vi "BellaBeamLine.vi"() -> ()   [LabVIEW 2020]
uses:
  StagingBeamline/Controls/eventtypdef1.ctl
  Shared/GUI_Template/GUI_master/tcp new data cluster.ctl
  Device Drivers/LEPS Interface/Filter_typdef.ctl
panel:
  in  "filter.var 2::15":T1=enum."OD1" caption="Filter Wheel"
  in  "filter.var 4::15":T1=enum."OD1" caption="Filter Wheel"
  in  "filter.var 5::15":T1=enum."OD1" caption="Filter Wheel"
  in  "filter.var 1::15":T1=enum."OD1" caption="Filter Wheel"
  in  "GUIdevice 15":string="71146 LEPS Interface"
  in  "stepsize::14":dbl=0.001 caption="Step Size" min=0.0 max=1.0 format="%.3f"
  in  "stepsize::12":dbl=0.001 caption="Step Size" min=0.0 max=1.0 format="%.3f"
  in  "stepsize::13":dbl=0.001 caption="Step Size" min=0.0 max=1.0 format="%.3f"
  in  "relativeMove.Axis 1pos::14":bool
  in  "relativeMove.Axis 1neg::14":bool
  in  "relativeMove.Axis 3pos::12":bool
  in  "relativeMove.Axis 3neg::12":bool
  in  "GUIdevice 14":string="BELLA_ESP_2"
  in  "relativeMove.Axis 2neg::14":bool
  in  "relativeMove.Axis 2pos::14":bool
  in  "relativeMove.Axis 3pos::14":bool
  in  "relativeMove.Axis 3neg::14":bool
  in  "GUIdevice 12":string="BellaESP"
  in  "relativeMove.Axis 1neg::12":bool
  in  "relativeMove.Axis 1pos::12":bool
  in  "relativeMove.Axis 2pos::12":bool
  in  "relativeMove.Axis 2neg::12":bool
  in  "GUIdevice 13":string="BELLA_ESP_M1"
  in  "relativeMove.Axis 1neg::13":bool
  in  "relativeMove.Axis 1pos::13":bool
  in  "relativeMove.Axis 2pos::13":bool
  in  "relativeMove.Axis 2neg::13":bool
  out "Boolean":bool
  in  "Dutch>>Magnet":bool caption="Mirror"
  out "GUIdevice 11":string="StagingImageLocation"
  out "GUIdevice 10":string="StagingImageLocation"
  out "GUIdevice 9":string="StagingTRA3"
  in  "GUIdevice 8":string="StagingTelescopePosition"
  in  "M5Cam>>Camera":bool caption="M5Cam"
  in  "M4Cam>>Camera":bool caption="M4Cam"
  in  "M2Cam>>Camera":bool caption="M2Cam"
  out "GUIdevice 7":string="StagingDelayStage"
  in  "DeviceControl":bool=TRUE
  in  "ignore interlock::6":bool=TRUE caption="ignore interlock"
  in  "GUIdevice 6":string="StagingInterlock"
  out "fire interlock::6":bool caption="Interlock"
  in  "GUIdevice 5":string="BellaSRS"
  out "fire::5":string
  in  "fire!!!":bool caption="fire"
  in  "Mode::5":bool
  out "GUIdevice 4":string="StagingImageLocation"
  in  "GUIdevice 3":string="StagingFocusPositionBeam2"
  in  "GUIdevice 2":string="StagingFocusPositionBeam1"
  out "XHairs":refnum<vi>[](array[refnum])
  out "device status::1":string="no scan"
  in  "GUIdevice 1":string="Staging1Wire"
  in  "M1Cam>>Camera":bool caption="M1Cam"
  in  "Bella_LP_Mode>>Camera":bool caption="Bella_LP_Mode"
  in  "stop":bool
  # "M5 X-Axis, LP Mode CAMS"
  # "M5 Y-Axis, M4 CAMS"
  # "M2 CAM"
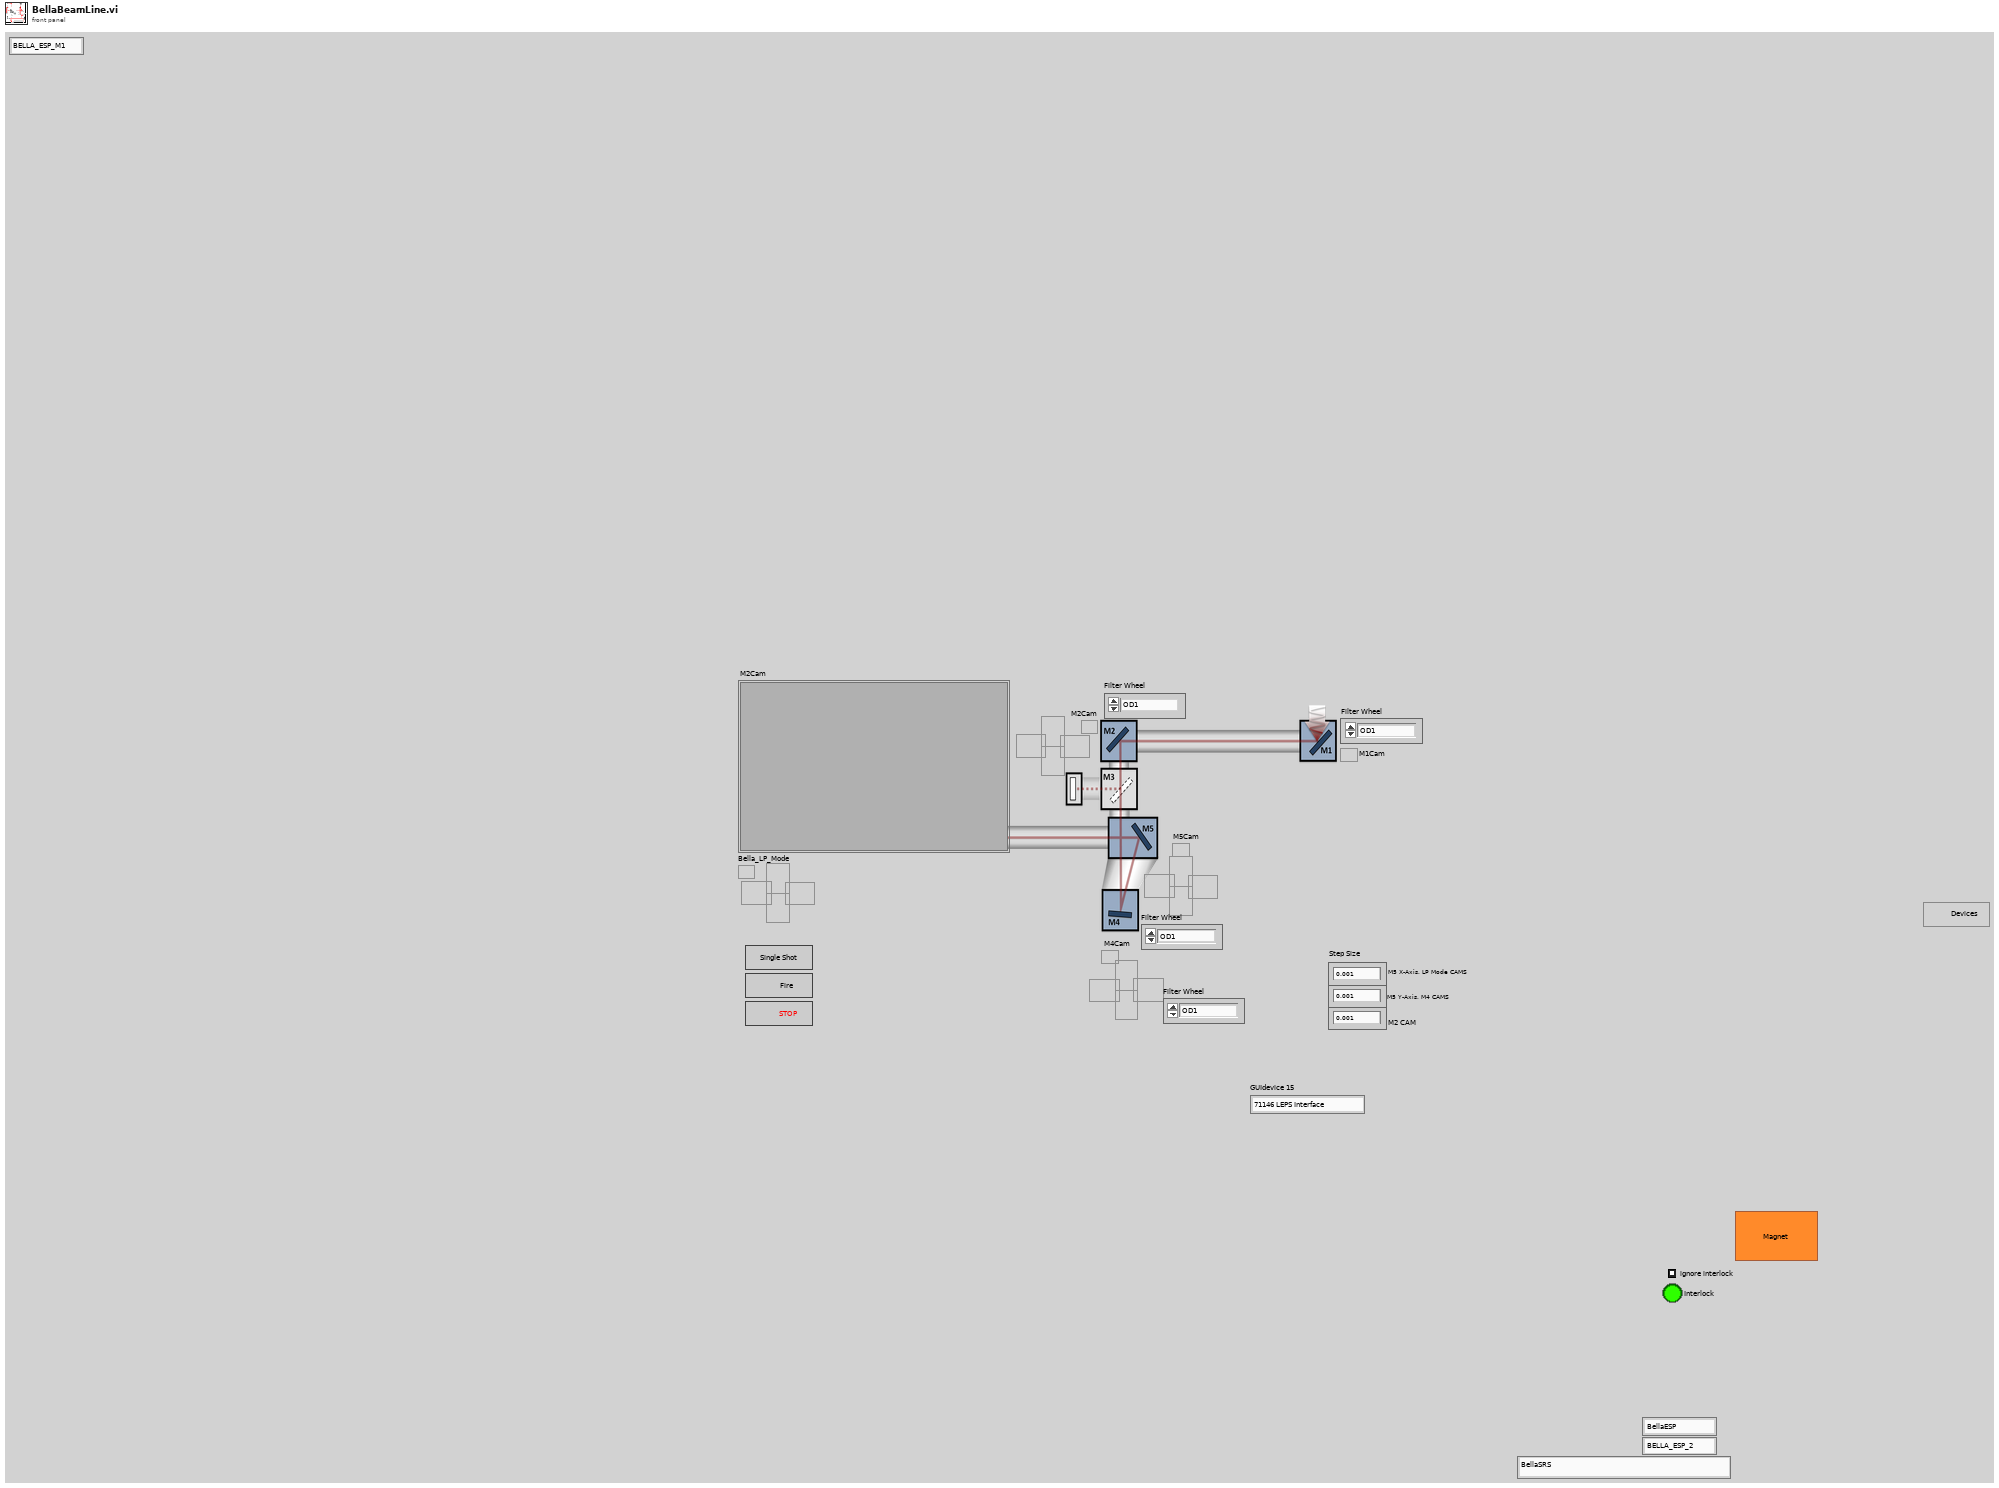
[diagram p1: front panel]
types:
  T1 = typedef "Filter_typdef.ctl" = enum16{"Moving/Unknown", "OD1", "OD2", "OD3", "OD4", "OD5", "Open(6)"}
  T2 = typedef "tcp new data cluster.ctl" = cluster{"EventEnum":enum16{"new data", "connection status update"}, "Device name":string}
  T3 = typedef "eventtypdef1.ctl" = cluster{"label":string, "Sub Panel":refnum<vi>, "CtlRef":refnum<vi>, "This VI":refnum<vi>}
  T4 = enum8{"Enabled", "Disabled", "Disabled and Grayed Out"}
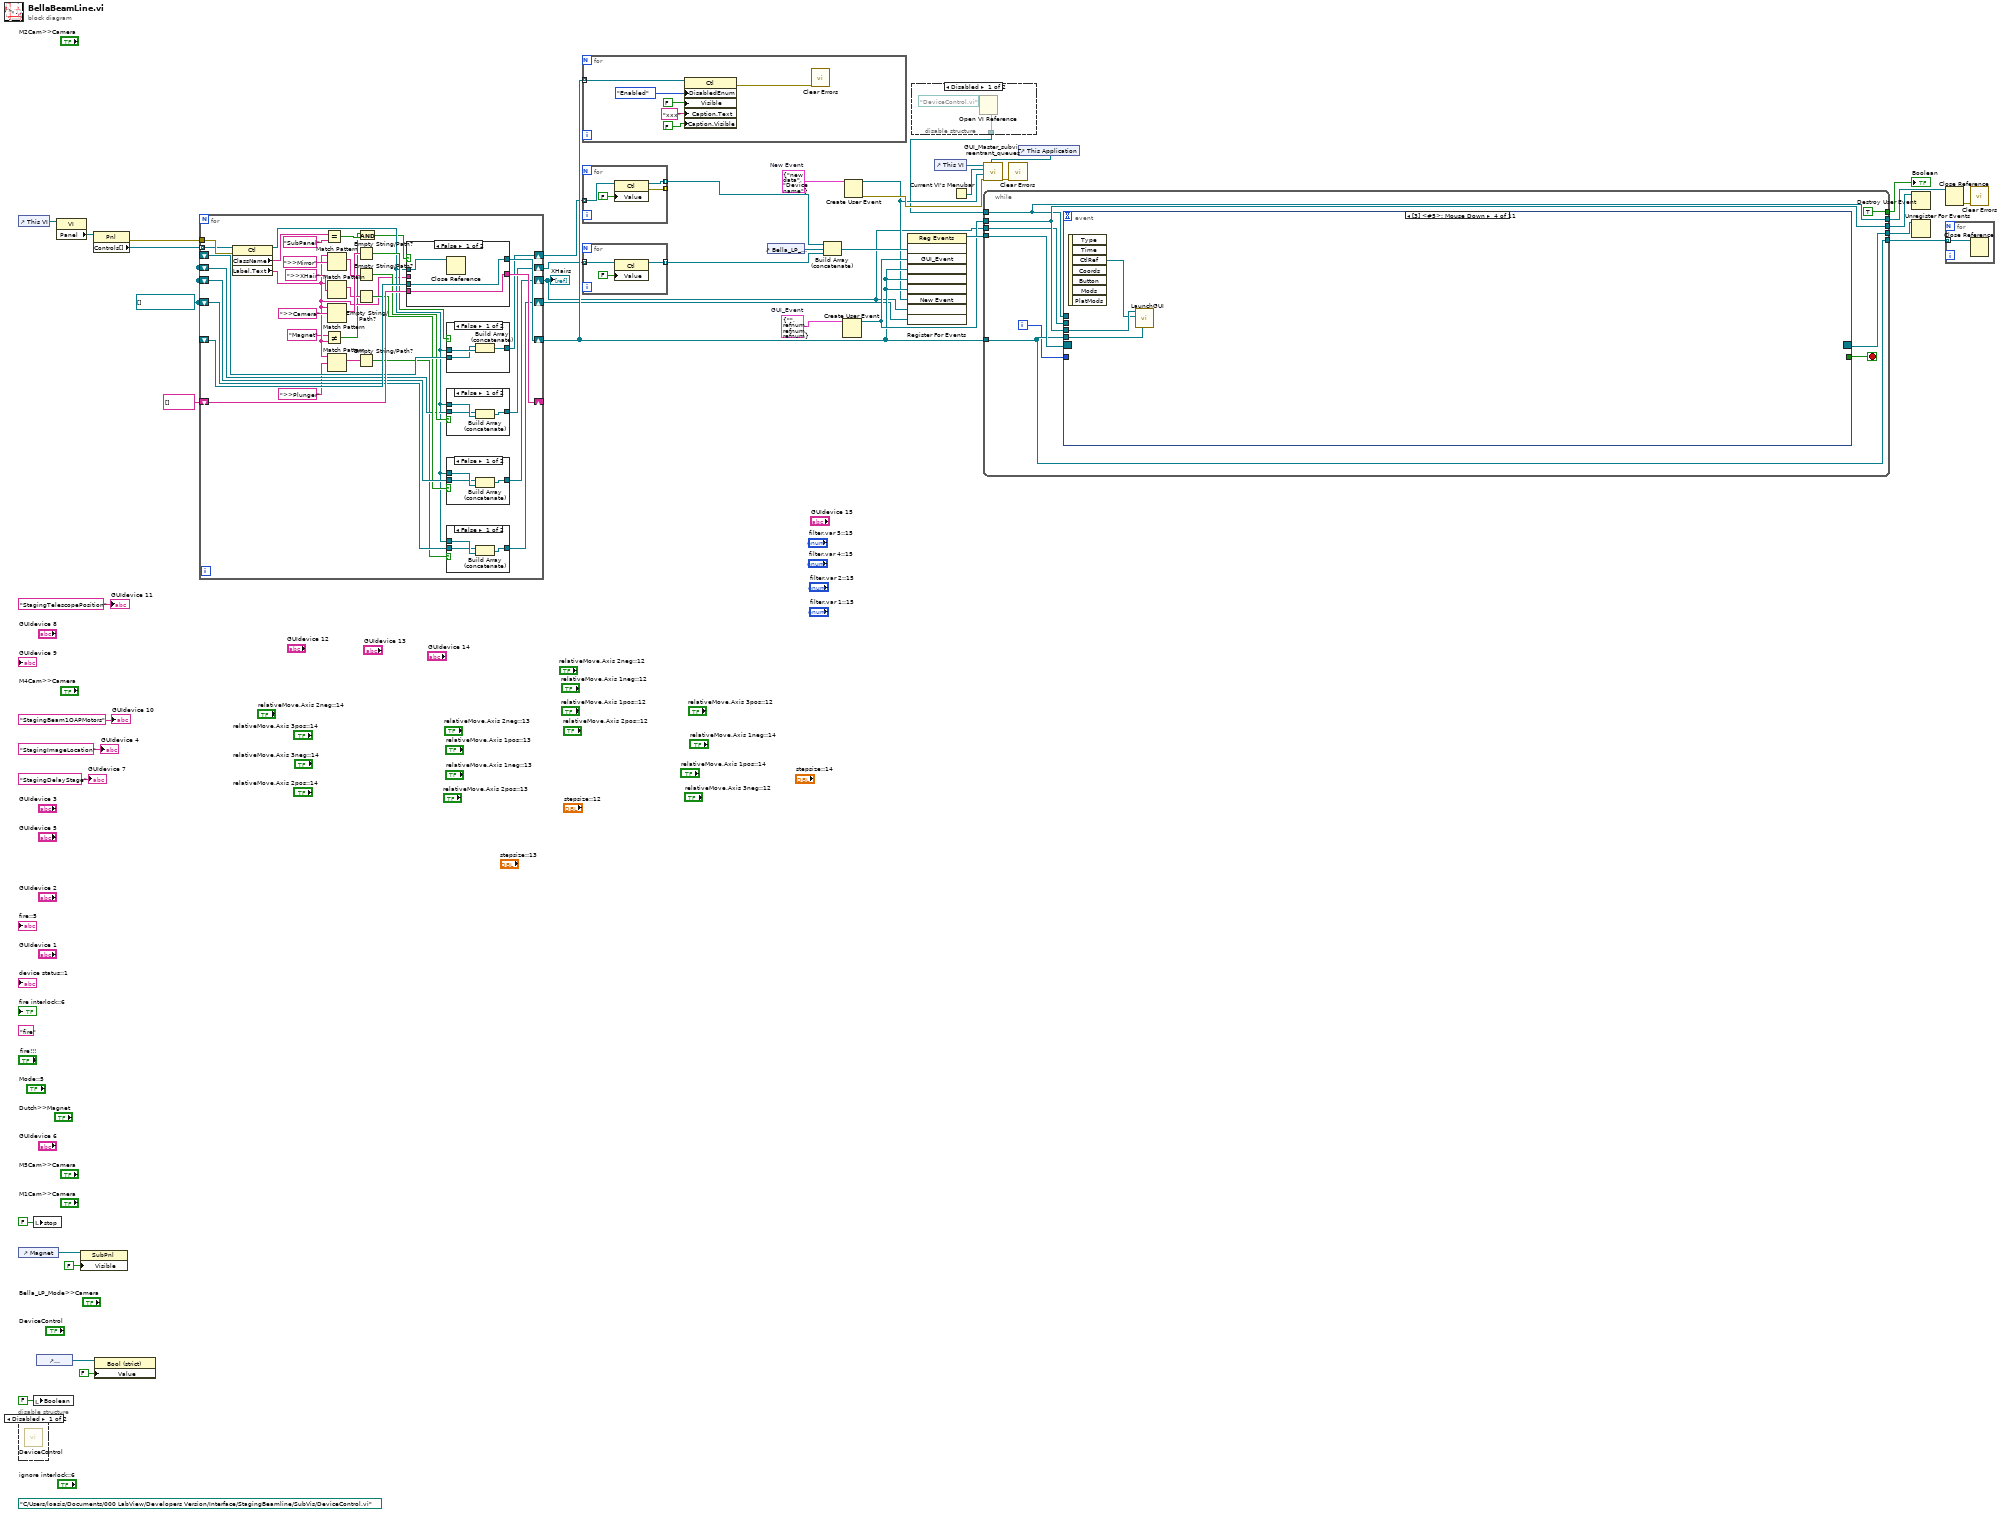
[diagram p0: block diagram]
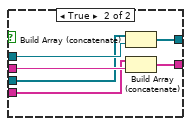
[diagram p8: hidden frame]
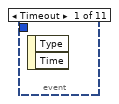
[diagram p9: hidden frame]
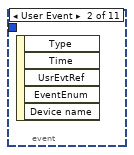
[diagram p10: hidden frame]
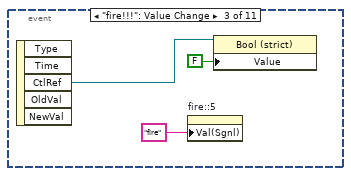
[diagram p11: hidden frame]
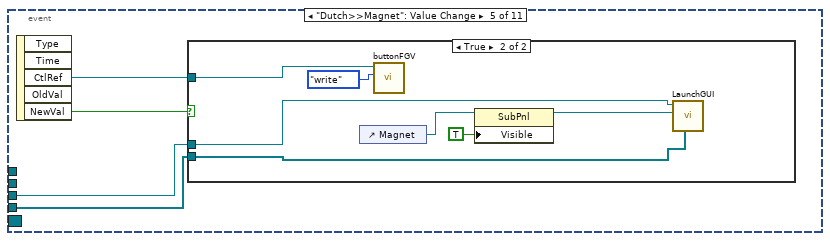
[diagram p12: hidden frame]
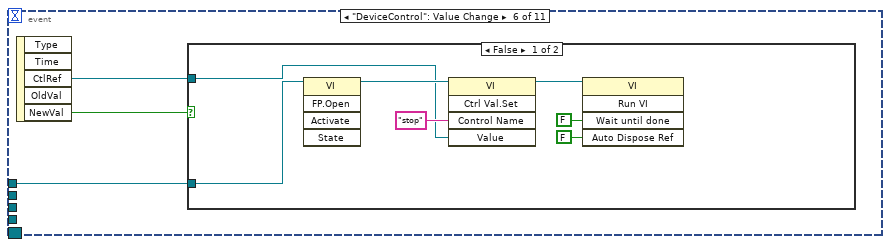
[diagram p14: hidden frame]
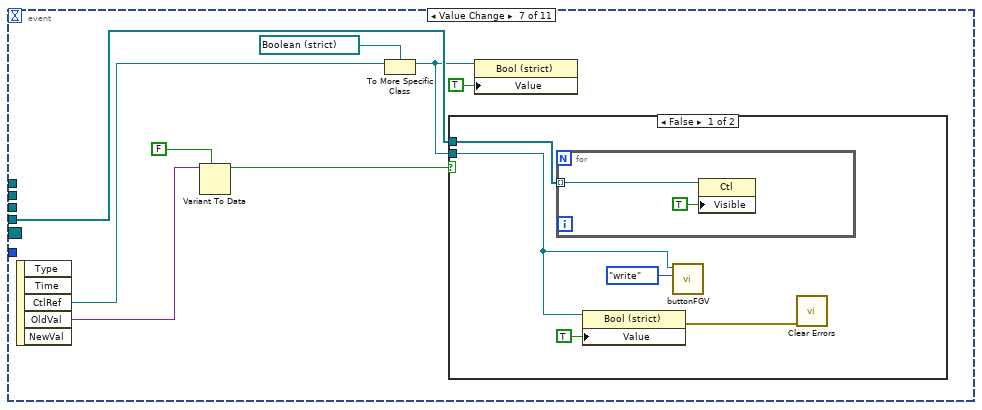
[diagram p16: hidden frame]
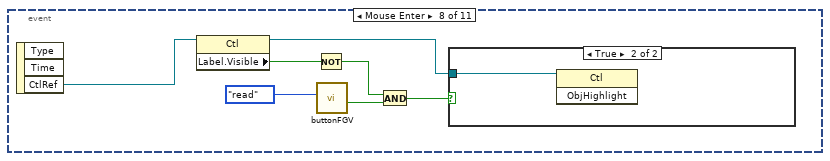
[diagram p18: hidden frame]
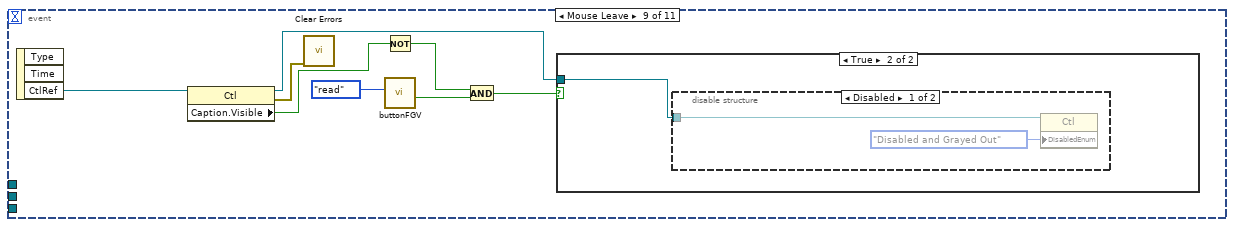
[diagram p20: hidden frame]
diagram:
  (unwired) path "C:/Users/loasis/Documents/000 LabView/Developers Version/Interface/StagingBeamline/SubVis/DeviceControl.vi" ("Path")
  (unwired) "fire" ("Value (Signaling)")
  w27 = T2 {"EventEnum"=enum."new data", "Device name"="Device name"}  # New Event
  w10 = refnum<vi>[] []
  w41 = T3 {"label"="", "Sub Panel"=refnum, "CtlRef"=refnum, "This VI"=refnum}  # GUI_Event
  n1 = control-ref of="This VI"() -> (w37:refnum<vi>)
  n2 = control-ref of="Magnet"() -> (w5:refnum<vi>)
  n3 = disable-structure shown="Disabled" {
    frame Disabled {
      n4 = call "DeviceControl.vi"() -> ()  [unwired: 11 in, 1 out]
    }
    frame Enabled {
    }
  }
  n5 = local write "stop"(FALSE ("stop")) -> ()
  n6 = local write "Boolean"(FALSE ("Boolean")) -> ()
  n7 = control-ref of="Dutch>>Magnet"() -> (w8:refnum<vi>)
  n8 = property class="VI"(reference=w37) -> ("Panel"=w36:refnum<vi>)  [unwired: 1 in, 2 out]
  n9 = property class="SubPnl"(reference=w5, "Visible"=FALSE) -> ()  [unwired: 1 in, 2 out]
  n10 = property class="Pnl"(reference=w36) -> (error out=w34:errorcluster, "Controls[]"=w35:refnum<vi>[])  [unwired: 1 in, 1 out]
  n11 = property class="Bool (strict)"(reference=w8, "Value"=FALSE) -> ()  [unwired: 1 in, 2 out]
  n12 = for {
    tunnel: w35 -> [w75] mode=indexing
    tunnel: w34 -> [w76]
    shift-right: [w72] -> _
    shift-left: string[] [] -> [w71]
    shift-right: [w70] -> w30
    shift-left: w10 -> [w69]
    shift-right: [w65] -> w23
    shift-left: w10 -> [w64]
    shift-right: [w63] -> w12
    shift-left: w10 -> [w62]
    shift-right: [w55] -> w18
    shift-left: w10 -> [w54]
    shift-right: [w51] -> w9
    shift-left: w10 -> [w52]
    n13 = property class="Ctl"(reference=w75, error in=w76) -> (reference out=w53:refnum<vi>, "ClassName"=w74:string, "Label.Text"=w47:string)  [unwired: 1 out]
    n14 = Equal?(x=w74, y="SubPanel") -> (x = y?=w45:bool)
    n15 = Not Equal?(x="Magnet", y=w47) -> (x != y?=w44:bool)
    n16 = Match Pattern(string=w47, regular expression=">>Mirror") -> (match substring=w57:string)  [unwired: 1 in, 3 out]
    n17 = Match Pattern(string=w47, regular expression=">>XHair") -> (match substring=w60:string)  [unwired: 1 in, 3 out]
    n18 = Match Pattern(string=w47, regular expression=">>Camera") -> (match substring=w67:string)  [unwired: 1 in, 3 out]
    n19 = Match Pattern(string=w47, regular expression=">>Plunger") -> (match substring=w49:string)  [unwired: 1 in, 3 out]
    n20 = Empty String/Path?(string/path=w67) -> (empty?=w66:bool)
    n21 = Empty String/Path?(string/path=w57) -> (empty?=w58:bool)
    n22 = Empty String/Path?(string/path=w60) -> (empty?=w59:bool)
    n23 = Empty String/Path?(string/path=w49) -> (empty?=w48:bool)
    n24 = And(x=w44, y=w45) -> (x .and. y?=w43:bool)
    n25 = case shown="False" w43 {
      tunnel: w53 -> [w95 w98]
      tunnel: w47 -> [_ w101]
      tunnel: [w94 w100] -> w72
      tunnel: w71 -> [w94 w99]
      tunnel: [w93 w97] -> w70
      tunnel: w69 -> [w93 w96]
      frame False {
        n26 = Close Reference(reference=w95) -> ()  [unwired: 1 in, 1 out]
      }
      frame True {
        n27 = Build Array (concatenate)(w96, w98) -> (w97:refnum<vi>[])
        n28 = Build Array (concatenate)(w99, w101) -> (w100:string[])
      }
    }
    n29 = case shown="False" w66 {
      tunnel: w53 -> [w91 _]
      tunnel: [w90 w92] -> w65
      tunnel: w64 -> [w89 w92]
      frame False {
        n30 = Build Array (concatenate)(w89, w91) -> (w90:refnum<vi>[])
      }
      frame True {
      }
    }
    n31 = case shown="False" w58 {
      tunnel: w53 -> [w83 _]
      tunnel: [w82 w84] -> w55
      tunnel: w54 -> [w81 w84]
      frame False {
        n32 = Build Array (concatenate)(w81, w83) -> (w82:refnum<vi>[])
      }
      frame True {
      }
    }
    n33 = case shown="False" w59 {
      tunnel: w53 -> [w87 _]
      tunnel: [w86 w88] -> w63
      tunnel: w62 -> [w85 w88]
      frame False {
        n34 = Build Array (concatenate)(w85, w87) -> (w86:refnum<vi>[])
      }
      frame True {
      }
    }
    n35 = case shown="False" w48 {
      tunnel: w53 -> [w79 _]
      tunnel: [w78 w80] -> w51
      tunnel: w52 -> [w77 w80]
      frame False {
        n36 = Build Array (concatenate)(w77, w79) -> (w78:refnum<vi>[])
      }
      frame True {
      }
    }
  }
  "XHairs" <- w12
  n37 = for {
    tunnel: w30 -> [w106] mode=indexing
    n38 = property class="Ctl"(reference=w106, "DisabledEnum"=T4."Enabled" ("Disabled"), "Visible"=FALSE, "Caption.Text"="xxx", "Caption.Visible"=FALSE ("Label.Visible")) -> (error out=w102:errorcluster)  [unwired: 1 in, 1 out]
    n39 = call <vilib>:"Clear Errors.vi"("error in (no error)"=w102) -> ()  [unwired: 5 in, 2 out]
  }
  n40 = for {
    tunnel: w23 -> [w111] mode=indexing
    tunnel: [w109] -> w22 mode=indexing
    tunnel: [w108] -> _ mode=indexing
    n41 = property class="Ctl"(reference=w111, "Value"=FALSE ("Visible")) -> (reference out=w109:refnum<vi>, error out=w108:errorcluster)  [unwired: 1 in]
  }
  n42 = for {
    tunnel: w18 -> [w114] mode=indexing
    tunnel: [w112] -> w17 mode=indexing
    n43 = property class="Ctl"(reference=w114, "Value"=FALSE ("Visible")) -> (reference out=w112:refnum<vi>)  [unwired: 1 in, 1 out]
  }
  n44 = control-ref of="Bella_LP_Mode>>Camera"() -> (w40:refnum<vi>)
  n45 = Build Array (concatenate)(w22, w40, w17) -> (w39:refnum<vi>[])
  n46 = Create User Event(user event datatype=w41) -> (user event=w31:refnum<user-event>)  [unwired: 1 in, 1 out]
  n47 = Create User Event(user event datatype=w27) -> (user event=w24:refnum<user-event>, error out=w28:errorcluster)  [unwired: 1 in]
  n48 = register-events(w39, w31, w30, w30, w30, w24, w12, w9) -> (reference out=w38:refnum<event-registration>)  [unwired: 2 in, 1 out]
  n49 = disable-structure shown="Disabled" {
    disable-tunnel: [w116 _] -> w19
    frame Disabled {
      n50 = Open VI Reference(vi path=path "DeviceControl.vi" ("Path")) -> (vi reference=w116:refnum<vi>)  [unwired: 5 in, 1 out]
    }
    frame Enabled {
    }
  }
  n51 = control-ref of="This VI"() -> (w25:refnum<vi>)
  n52 = Current VI's Menubar() -> (w26:refnum<k9>)
  n53 = while {
    tunnel: w31 -> [w124]
    tunnel: [w124] -> w42
    tunnel: w38 -> [w123]
    tunnel: w30 -> [w122]
    tunnel: [w122] -> w32
    tunnel: w12 -> [w120]
    tunnel: [w119] -> w21
    tunnel: w19 -> [w119]
    tunnel: [w118] -> w11
    tunnel: [TRUE] -> w3
    i -> [w121]
    stop <- w125 stop-if-true
    n54 = event shown="[3] <#5>: Mouse Down" {
      selector: w123 -> [_ _ _ _ _ _ _ _ _ _ _]
      dyn-events: [_ _ _ _ _ _ _ _ _ _ _] -> w118
      timeout: _ -> [_ _ _ _ _ _ _ _ _ _ _]
      tunnel: [_ _ _ _ _ _ _ _ _ _ "stop"] -> w125
      tunnel: w124 -> [_ _ _ w131 w135 _ _ _ _ _ w219]
      tunnel: w122 -> [_ _ _ w130 w133 _ w160 _ _ _ _]
      tunnel: w121 -> [_ _ _ _ _ _ _ _ _ _ _]
      tunnel: w120 -> [_ _ _ _ _ _ _ _ _ _ _]
      tunnel: w119 -> [_ _ _ _ _ w143 _ _ _ _ _]
      event Timeout {
        n55 = event-data() -> ()  [unwired: 1 in, 2 out]
      }
      event User Event {
        n56 = event-data() -> ()  [unwired: 1 in, 5 out]
      }
      event "fire!!!": Value Change {
        n57 = event-data() -> ("CtlRef"=w127:refnum<vi>)  [unwired: 1 in, 4 out]
        n58 = property on="fire::5" class="Str"("Val(Sgnl)"="fire" ("fire::5")) -> ()  [unwired: 2 in, 2 out]
        n59 = property class="Bool (strict)"(reference=w127, "Value"=FALSE) -> ()  [unwired: 1 in, 2 out]
      }
      event Mouse Down {
        n60 = event-data() -> ("CtlRef"=w129:refnum<vi>)  [unwired: 1 in, 6 out]
        n61 = call "LaunchGUI.vi"("Array"=w130, "CtlRef"=w129, "User Event in"=w131) -> ()  [unwired: 9 in]
      }
      event "Dutch>>Magnet": Value Change {
        n62 = event-data() -> ("CtlRef"=w134:refnum<vi>, "NewVal"=w132:bool)  [unwired: 1 in, 3 out]
        n63 = case shown="True" w132 {
          tunnel: w135 -> [_ w142]
          tunnel: w134 -> [_ w140]
          tunnel: w133 -> [_ w139]
          frame False {
          }
          frame True {
            n64 = control-ref of="Magnet"() -> (w138:refnum<vi>)
            n65 = call "buttonFGV.vi"("command"=enum16{"read", "write"}."write", "Boolean in"=w140) -> ()  [unwired: 7 in, 3 out]
            n66 = property class="SubPnl"(reference=w138, "Visible"=TRUE) -> (reference out=w137:refnum<vi>)  [unwired: 1 in, 1 out]
            n67 = call "LaunchGUI.vi"("Array"=w139, "CtlRef"=w137, "User Event in"=w142) -> ()  [unwired: 9 in]
          }
        }
      }
      event "DeviceControl": Value Change {
        n68 = event-data() -> ("CtlRef"=w145:refnum<vi>, "NewVal"=w144:bool)  [unwired: 1 in, 3 out]
        n69 = case shown="False" w144 {
          tunnel: w143 -> [w152 _]
          tunnel: w145 -> [w146 _]
          frame False {
            n70 = invoke class="VI" method="FP.Open"(reference=w152) -> (reference out=w149:refnum<vi>)  [unwired: 4 in, 4 out]
            n71 = invoke class="VI" method="Ctrl Val.Set"(reference=w149, "Control Name"="stop", "Value"=w146) -> (reference out=w148:refnum<vi>)  [unwired: 2 in, 4 out]
            n72 = invoke class="VI" method="Run VI"(reference=w148, "Wait until done"=FALSE ("Wait Until Done"), "Auto Dispose Ref"=FALSE ("Auto Dispose Reference")) -> ()  [unwired: 2 in, 5 out]
          }
          frame True {
          }
        }
      }
      event Value Change {
        n73 = event-data() -> ("CtlRef"=w155:refnum<vi>, "OldVal"=w158:variant)  [unwired: 1 in, 3 out]
        n74 = Variant To Data(type=FALSE, Variant=w158) -> (data=w156:bool)  [unwired: 1 in, 1 out]
        n75 = To More Specific Class(target class=refnum<vi> refnum ("Boolean in"), reference=w155) -> (specific class reference=w154:refnum<vi>)  [unwired: 1 in, 1 out]
        n76 = case shown="False" w156 {
          tunnel: w160 -> [w164 _]
          tunnel: w154 -> [w161 _]
          frame False {
            n77 = for {
              tunnel: w164 -> [w166] mode=indexing
              n78 = property class="Ctl"(reference=w166, "Visible"=TRUE) -> ()  [unwired: 1 in, 2 out]
            }
            n79 = property class="Bool (strict)"(reference=w161, "Value"=TRUE) -> (error out=w162:errorcluster)  [unwired: 1 in, 1 out]
            n80 = call "buttonFGV.vi"("command"=enum16{"read", "write"}."write", "Boolean in"=w161) -> ()  [unwired: 7 in, 3 out]
            n81 = call <vilib>:"Clear Errors.vi"("error in (no error)"=w162) -> ()  [unwired: 5 in, 2 out]
          }
          frame True {
          }
        }
        n82 = property class="Bool (strict)"(reference=w154, "Value"=TRUE) -> ()  [unwired: 1 in, 2 out]
      }
      event Mouse Enter {
        n83 = event-data() -> ("CtlRef"=w173:refnum<vi>)  [unwired: 1 in, 2 out]
        n84 = property class="Ctl"(reference=w173) -> (reference out=w172:refnum<vi>, "Label.Visible"=w171:bool)  [unwired: 1 in, 1 out]
        n85 = Not(x=w171) -> (.not. x?=w170:bool)
        n86 = call "buttonFGV.vi"("command"=enum16{"read", "write", "clear"}."read" ("Enum")) -> ("select subPanel"=w169:bool)  [unwired: 8 in, 2 out]
        n87 = And(x=w170, y=w169) -> (x .and. y?=w168:bool)
        n88 = case shown="True" w168 {
          tunnel: w172 -> [_ w175]
          frame False {
          }
          frame True {
            n89 = invoke class="Ctl" method="ObjHighlight"(reference=w175) -> ()  [unwired: 2 in, 3 out]
          }
        }
      }
      event Mouse Leave {
        n90 = event-data() -> ("CtlRef"=w182:refnum<vi>)  [unwired: 1 in, 2 out]
        n91 = property class="Ctl"(reference=w182) -> (reference out=w181:refnum<vi>, error out=w176:errorcluster, "Caption.Visible"=w180:bool)  [unwired: 1 in]
        n92 = call <vilib>:"Clear Errors.vi"("error in (no error)"=w176) -> ()  [unwired: 5 in, 2 out]
        n93 = Not(x=w180) -> (.not. x?=w179:bool)
        n94 = call "buttonFGV.vi"("command"=enum16{"read", "write", "clear"}."read" ("Enum")) -> ("select subPanel"=w178:bool)  [unwired: 8 in, 2 out]
        n95 = And(x=w179, y=w178) -> (x .and. y?=w177:bool)
        n96 = case shown="True" w177 {
          tunnel: w181 -> [_ w184]
          frame False {
          }
          frame True {
            n97 = disable-structure shown="Disabled" {
              disable-tunnel: w184 -> [w185 _]
              frame Disabled {
                n98 = property class="Ctl"(reference=w185, "DisabledEnum"=T4."Disabled and Grayed Out" ("Disabled")) -> ()  [unwired: 1 in, 2 out]
              }
              frame Enabled {
              }
            }
          }
        }
      }
      event User Event {
        n99 = event-data() -> ("CtlRef"=w196:refnum<vi>, "Sub Panel"=w199:refnum<vi>, "This VI"=w198:refnum<vi>, "label"=w195:string)  [unwired: 1 in, 3 out]
        n100 = Match Pattern(string=w195, regular expression=">>" ("search string")) -> (before substring=w193:string, after substring=w192:string)  [unwired: 1 in, 2 out]
        n101 = Equal?(x=w192, y="new vi") -> (x = y?=w189:bool)
        n102 = Equal?(x=w193, y="vi closed" ("label")) -> (x = y?=w190:bool)
        n103 = case shown="True" w190 {
          tunnel: w196 -> [_ w200]
          frame False {
          }
          frame True {
            n104 = property class="Bool (strict)"(reference=w200, "Value"=FALSE) -> (error out=w202:errorcluster)  [unwired: 1 in, 1 out]
            n105 = call <vilib>:"Clear Errors.vi"("error in (no error)"=w202) -> ()  [unwired: 5 in, 2 out]
          }
        }
        n106 = Not(x=w189) -> (.not. x?=w188:bool)
        n107 = And(x=w190, y=w188) -> (x .and. y?=w187:bool)
        n108 = case shown="True" w187 {
          tunnel: w199 -> [_ w209]
          tunnel: w198 -> [_ w208]
          frame False {
          }
          frame True {
            w204 = FALSE ("Visible")
            n109 = invoke class="SubPnl" method="Remove VI"(reference=w209) -> (reference out=w207:refnum<vi>, error out=w205:errorcluster)  [unwired: 2 in, 1 out]
            n110 = disable-structure shown="Enabled" {
              disable-tunnel: w208 -> [w212 _]
              disable-tunnel: [w211 w213] -> w206
              disable-tunnel: w205 -> [w210 w213]
              frame Disabled {
                n111 = Close Reference(reference=w212, error in (no error)=w210) -> (error out=w211:errorcluster)
              }
              frame Enabled {
              }
            }
            n112 = property class="SubPnl"(reference=w207, error in=w206, "Visible"=w204, "Label.Visible"=w204) -> (error out=w203:errorcluster)  [unwired: 1 out]
            n113 = call <vilib>:"Clear Errors.vi"("error in (no error)"=w203) -> ()  [unwired: 5 in, 2 out]
          }
        }
      }
      event "stop": Value Change {
        n114 = event-data() -> ("CtlRef"=w221:refnum<vi>)  [unwired: 1 in, 4 out]
        n115 = property on="DeviceControl" class="Bool (strict)"("Val(Sgnl)"=TRUE ("Value (Signaling)")) -> (error out=w214:errorcluster)  [unwired: 2 in, 1 out]
        n116 = Generate User Event(user event=w219, event data cluster=T3 {"label"="stop", "Sub Panel"=refnum, "CtlRef"=refnum, "This VI"=refnum} ("event data")) -> (error out=w217:errorcluster)  [unwired: 2 in, 1 out]
        n117 = call <userlib>:"Wait (ms)__ogtk.vi"("error in (no error)"=w217, "milliseconds to wait"=u32 1000) -> ()  [unwired: 8 in, 2 out]
        n118 = property class="Bool (strict)"(reference=w221, error in=w214, "Value"=FALSE) -> ()  [unwired: 2 out]
      }
    }
  }
  "Boolean" <- w3
  n119 = control-ref of="This Application"() -> (w1:refnum<vi>)
  n120 = call "GUI_Master_subvi_reentrant_queues.vi"("This Application"=w1, "error in (no error)"=w28, "tcp data event"=w24, "Caller menu reference"=w26, "Caller VI ref"=w25) -> ("error out"=w29:errorcluster)  [unwired: 6 in]
  n121 = call <vilib>:"Clear Errors.vi"("error in (no error)"=w29) -> ()  [unwired: 5 in, 2 out]
  n122 = Destroy User Event(user event=w42) -> ()  [unwired: 1 in, 1 out]
  n123 = Unregister For Events(event registration refnum=w11) -> ()  [unwired: 1 in, 1 out]
  n124 = Close Reference(reference=w21) -> (error out=w20:errorcluster)  [unwired: 1 in]
  n125 = for {
    tunnel: w32 -> [w223] mode=indexing
    n126 = Close Reference(reference=w223) -> ()  [unwired: 1 in, 1 out]
  }
  n127 = call <vilib>:"Clear Errors.vi"("error in (no error)"=w20) -> ()  [unwired: 5 in, 2 out]
  "GUIdevice 4" <- "StagingImageLocation" ("GUIdevice 4")
  "GUIdevice 7" <- "StagingDelayStage" ("GUIdevice 7")
  "GUIdevice 10" <- "StagingBeam1OAPMotors" ("GUIdevice 4")
  "GUIdevice 11" <- "StagingTelescopePosition" ("GUIdevice 4")
